vi "Write Time and Date Info.vi"(6 "错误输入":cluster{"状态":bool, "代码":i32, "源":string}, 9 "文件引用句柄输入":refnum<file>) -> (0 "错误输出":cluster{"状态":bool, "代码":i32, "源":string}, 3 "文件引用句柄输出":refnum<file>)   [LabVIEW 2012]
doc: "本VI按照日期和时间自动生成一个字符串，并打开以该字符串为名称的文件。包含一个正弦波和一个方波的数组被转换为制表符分隔的字符串，并写入文件。然后关闭文件。"
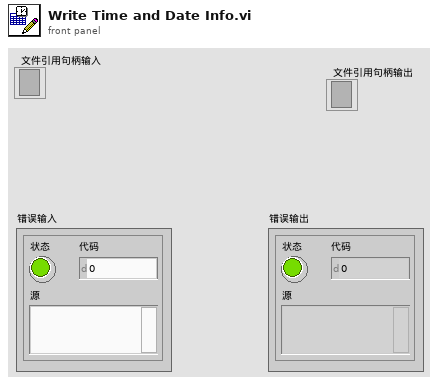
[diagram p1: front panel]
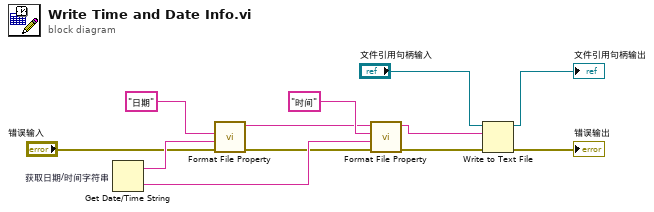
[diagram p0: block diagram]
diagram:
  n1 = Get Date/Time String "获取日期/时间字符串"() -> (date string=w11:string, time string=w8:string)  [unwired: 3 in]
  n2 = call "Format File Property.vi"("错误输入"="错误输入", "文件属性值"=w11, "文件属性名称"="日期") -> ("错误输出"=w7:cluster{"状态":bool, "代码":i32, "源":string}, "字符串输出"=w9:string)  [unwired: 7 in]
  n3 = call "Format File Property.vi"("错误输入"=w7, "文件属性值"=w8, "文件属性名称"="时间", "字符串输入"=w9) -> ("错误输出"=w2:cluster{"状态":bool, "代码":i32, "源":string}, "字符串输出"=w1:string)  [unwired: 6 in]
  n4 = Write to Text File ("写入文本文件")(file (use dialog)="文件引用句柄输入", text=w1, error in=w2) -> (refnum out=→"文件引用句柄输出":refnum<file>, error out=→"错误输出":errorcluster)  [unwired: 1 in, 1 out]
